vi "DrivePID.vi"(11 "Time Delay Milli":u32) -> ()   [LabVIEW 2012]
uses:
  System Set Points and States.vi
  <vilib>/addons/control/pid/pid.llb/PID (DBL).vi
  <vilib>/Rock Robotics/WPI/RobotDrive/WPI_RobotDriveGetSetRefNum.vi
  <vilib>/addons/control/pid/NI_PID_pid.lvlib
panel:
  out "Stable":bool
  out "Speed Error":cluster{dbl, dbl, dbl[]}(graph)
  out "Output 2":dbl
  out "Output":dbl
  in  "Graph time interval  in seconds":dbl
  out "Drive Speed":cluster{dbl, dbl, dbl[]}(graph)
  out "RPM Error":dbl
  out "Encoder Speed":dbl
  in  "D":dbl=0.001
  in  "I":dbl=0.05
  in  "P":dbl=0.0025 step=0.001
  out "Encoder Set Speed":dbl
  # "These Work\n0.0025\n0.05\n0.001"
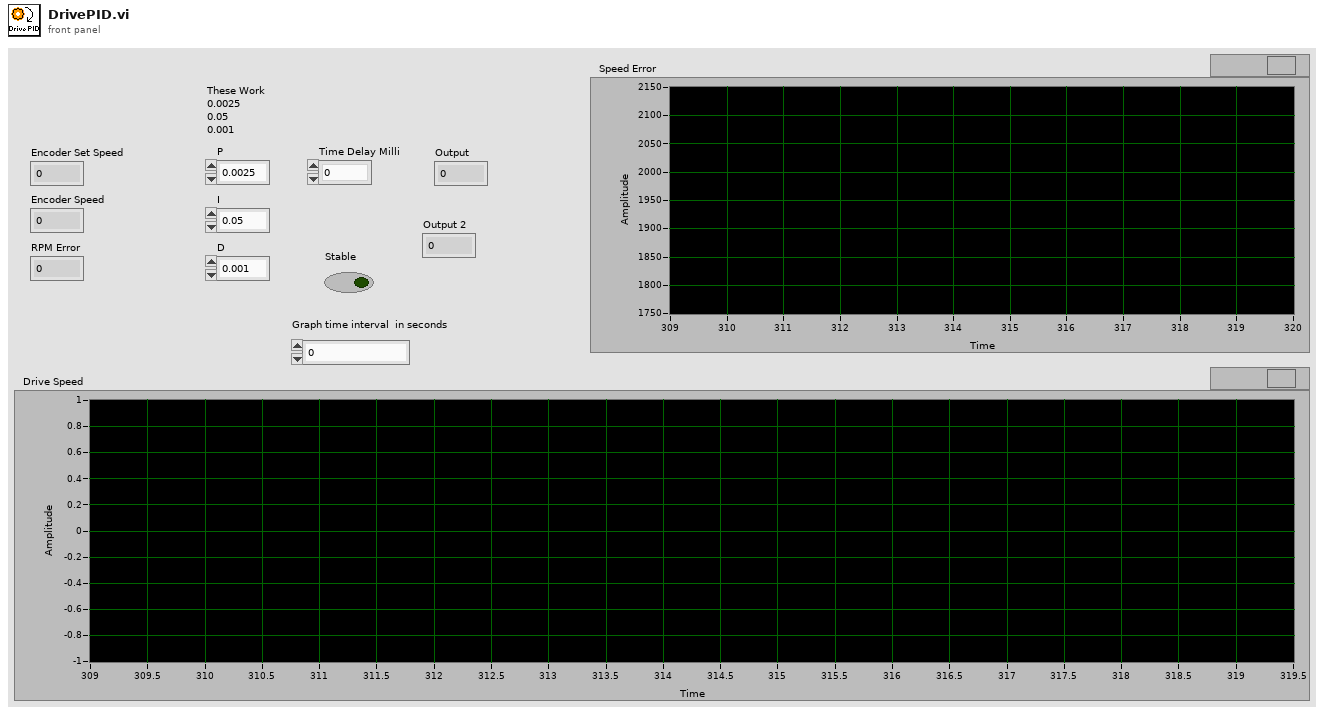
[diagram p1: front panel]
types:
  T1 = typedef "WPI_EncoderDevRef.ctl" = cluster{"DevStatus":errorcluster, "EncoderIndex":T2, "CounterIndex":T3, "DistancePerCount":dbl, "Decoding Type":T4}
  T2 = typedef "FPGA_EncoderIdx.ctl" = enum8{"Enc 0", "Enc 1", "Enc 2", "Enc 3", "Invalid"}
  T3 = typedef "FPGA_CounterCtrSystemIndex.ctl" = enum8{"Ctr 0", "Ctr 1", "Ctr 2", "Ctr 3", "Ctr 4", "Ctr 5", "Ctr 6", "Ctr 7", "Invalid"}
  T4 = typedef "WPI_EncoderType.ctl" = enum16{"1x", "2x", "4x"}
  T5 = typedef "WPI_RobotDriveDevRef.ctl" = cluster{"DevStatus":errorcluster, "Motors[]":T6[], "Square Inputs":bool, "Max Output":dbl, "Isochronous":bool}
  T6 = typedef "WPI_MotorControlDeviceRef.ctl" = cluster{"DeviceStatus":errorcluster, "Type":enum16{"PWM", "CAN"}, "PWM":cluster{"Digital Module":T7, "PWM Channel":T8, "DeadBand":T9}, "CAN":cluster{"Device Number":u8, "Control Mode":T10, "Semaphore":T11, "Max Vout":dbl}, "Invert":bool, "TransformRef":T12, "InvTransformRef":T12}
  T7 = typedef "FPGA_TypedefDigitalModule.ctl" = enum16{"Digital Module 1", "Digital Module 2"}
  T8 = typedef "FPGA_DIOPWMChannel.ctl" = enum8{"PWM 1", "PWM 2", "PWM 3", "PWM 4", "PWM 5", "PWM 6", "PWM 7", "PWM 8", "PWM 9", "PWM 10", "Invalid"}
  T9 = typedef "WPI_PWMDeadband.ctl" = cluster{"Name":string, "maxPositivePwm":i32, "minPositivePwm":i32, "centerPwm":i32, "maxNegativePwm":i32, "minNegativePwm":i32, "angularRange":u16}
  T10 = typedef "WPI_CANJaguar_ControlMode.ctl" = enum8{"Percent VBus", "Current", "Speed", "Position", "Voltage"}
  T11 = typedef "Semaphore RefNum" = refnum<k1>
  T12 = typedef "WPI_PWMTransform_ConPane.ctl" = refnum<vi>
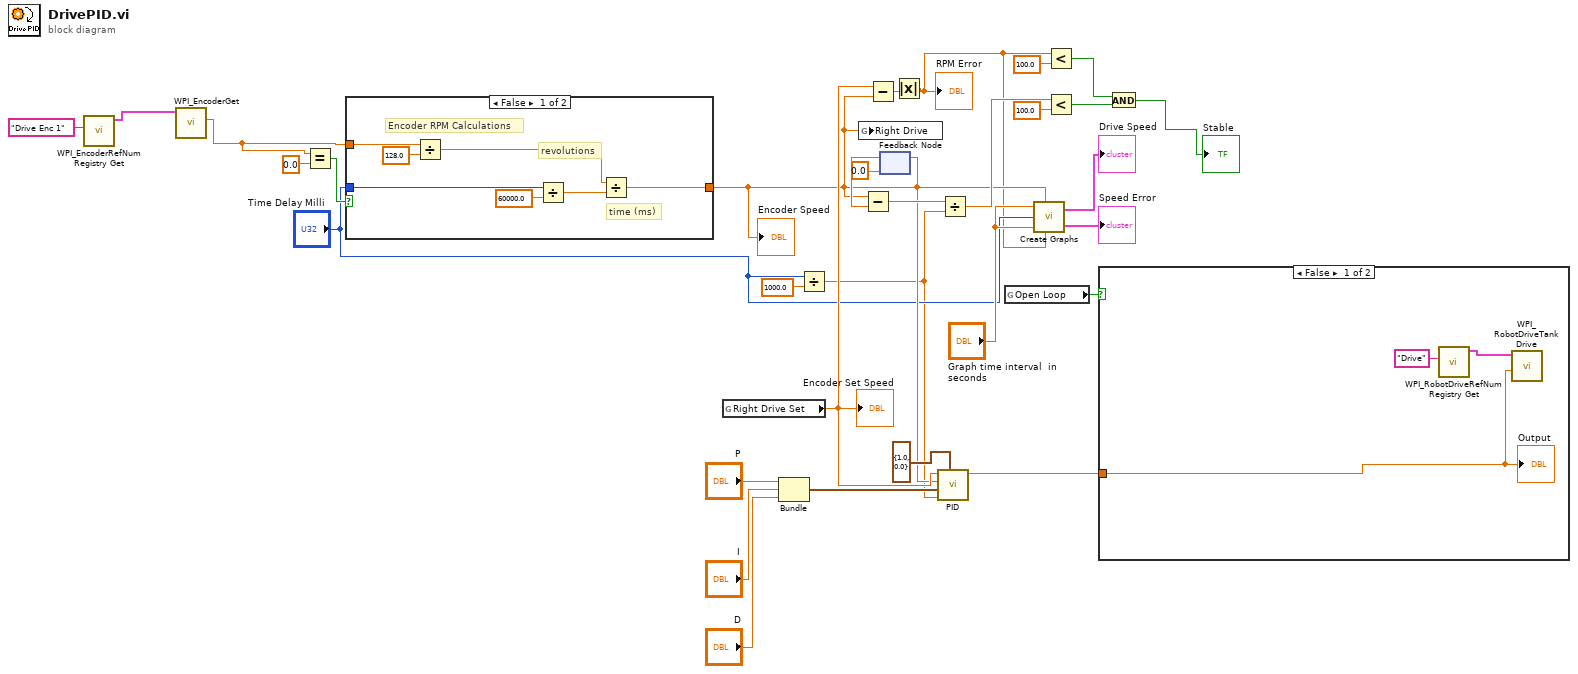
[diagram p0: block diagram]
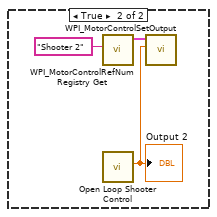
[diagram p2: hidden frame]
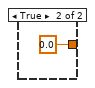
[diagram p3: hidden frame]
diagram:
  n1 = call <vilib>:"WPI_EncoderRefNum Registry Get.vi"("refnum name"="Drive Enc 1") -> ("EncoderDevRef"=w2:T1)  [unwired: 9 in, 1 out]
  n2 = call <vilib>:"WPI_EncoderGet.vi"("EncoderDevRef"=w2) -> ("Distance"=w3:dbl)  [unwired: 5 in, 5 out]
  n3 = Equal?(x=w3, y=0.0) -> (x = y?=w24:bool)
  n4 = case shown="False" w24 {
    tunnel: [w38 0.0] -> w11
    tunnel: w3 -> [w37 _]
    tunnel: "Time Delay Milli" -> [w35 _]
    frame False {
      # "time (ms)"
      # "revolutions"
      # "Encoder RPM Calculations"
      n5 = Divide(x=w37, y=128.0) -> (x/y=w36:dbl)
      n6 = Divide(x=w35, y=60000.0) -> (x/y=w33:dbl)
      n7 = Divide(x=w36, y=w33) -> (x/y=w38:dbl)
    }
    frame True {
    }
  }
  "Encoder Speed" <- w11
  n8 = global read "System Set Points and States.vi" "Right Drive Set"() -> (w26:dbl)
  "Encoder Set Speed" <- w26
  n9 = Bundle("P"="P", "I"="I", "D"="D") -> (w27:cluster{"P":dbl, "I":dbl, "D":dbl})  [unwired: 1 in]
  n10 = Divide(x="Time Delay Milli", y=1000.0) -> (x/y=w7:dbl)
  n11 = global write "System Set Points and States.vi" "Right Drive"(w11) -> ()
  n12 = Subtract(x=w26, y=w11) -> (x-y=w5:dbl)
  n13 = feedback-in #1(w11) -> ()
  n14 = feedback #1(0.0) -> (w21:dbl)
  n15 = Subtract(x=w11, y=w21) -> (x-y=w20:dbl)
  n16 = Absolute Value(x=w5) -> (abs(x)=w4:dbl)
  "RPM Error" <- w4
  n17 = call-poly <vilib>:"PID.vi"("output range"=cluster{"output high":dbl, "output low":dbl} {"output high"=1.0, "output low"=0.0}, "dt (s)"=w7, "PID gains"=w27, "process variable"=w11, "setpoint"=w26) -> ("output"=w23:dbl)  [unwired: 5 in, 1 out]
  n18 = Divide(x=w20, y=w7) -> (x/y=w19:dbl)
  n19 = global read "System Set Points and States.vi" "Open Loop"() -> (w22:bool)
  n20 = call "Create Graphs.vi"("Speed Graph Time"="Graph time interval  in seconds", "Speed"=w11, "Time Delay"="Time Delay Milli", "Error Graph Time"="Graph time interval  in seconds", "Error"=w4) -> ("Speed"=→"Drive Speed":cluster{dbl, dbl, dbl[]}, "Error"=→"Speed Error":cluster{dbl, dbl, dbl[]})
  n21 = Less?(x=w4, y=100.0) -> (x < y?=w15:bool)
  n22 = Less?(x=w19, y=100.0) -> (x < y?=w17:bool)
  n23 = case shown="False" w22 {
    tunnel: w23 -> [w40 _]
    frame False {
      n24 = call <vilib>:"WPI_RobotDriveRefNum Registry Get.vi"("refnum name"="Drive") -> ("RobotDriveDevRef"=w42:T5)  [unwired: 9 in, 1 out]
      n25 = call <vilib>:"WPI_RobotDriveTankDrive.vi"("Right axis value"=w40, "RobotDriveDevRef"=w42) -> ()  [unwired: 7 in, 3 out]
      "Output" <- w40
    }
    frame True {
      n26 = call <vilib>:"WPI_MotorControlRefNum Registry Get.vi"("refnum name"="Shooter 2") -> ("MotorControlDevRef"=w44:T6)  [unwired: 9 in, 1 out]
      n27 = call "Open Loop Shooter Control.vi"() -> ("Open Loop PWM"=w43:dbl)  [unwired: 11 in]
      "Output 2" <- w43
      n28 = call <vilib>:"WPI_MotorControlSetOutput.vi"("Output"=w43, "MotorControlDevRef"=w44) -> ()  [unwired: 7 in, 3 out]
    }
  }
  n29 = And(x=w15, y=w17) -> (x .and. y?=→"Stable":bool)
